vi "ONL.vi"(0 "System no.":i32=1 min=1 max=4 step=1, 2 "Channels to command":string[](array[string]), 3 "Online status":bool=TRUE, 4 "Online status (Array)":bool[](array[boolean]), 5 "error in":errorcluster) -> (19 "error out":errorcluster)   [LabVIEW 2020]
doc: "Switches system online (TRUE) or offline (FALSE). GCS 1.0: Online status is valid for all channels/axes of the system. GCS 2.0: Online status is channel specific.\n\nE-516: Channels to command and Online status (Array) are not valid, use Online status instead to set online status for all channels/axes.\n\nE-517, E-518: Online status is not valid. Use Channels to command and Online status (Array) instead."
uses:
  Communication.llb/Global1.vi
panel:
  # "Switches system online (TRUE) or offline (FALSE). GCS 1.0: Online status is valid for all channels/axes\nof the system. GCS 2.0: Online status is channel specific."
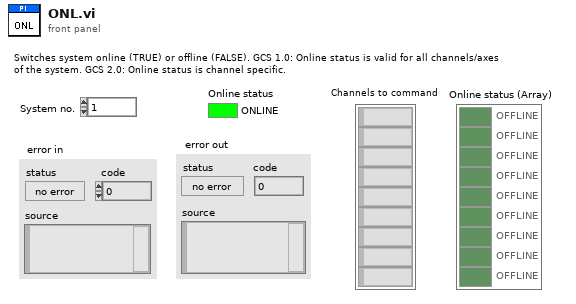
[diagram p1: front panel]
types:
  T1 = typedef "Syntax.ctl" = enum16{"GCS 1.0", "GCS 2.0", "GCS 3.0"}
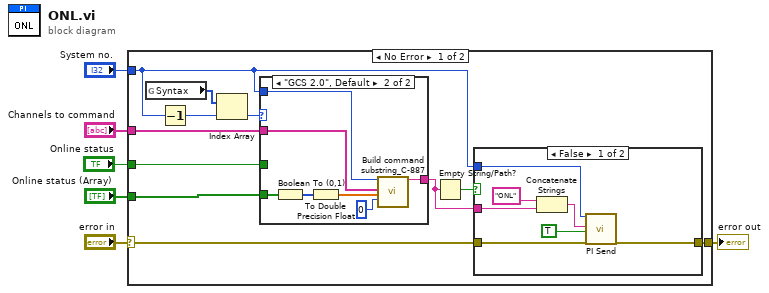
[diagram p0: block diagram]
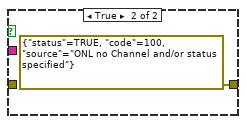
[diagram p2: hidden frame]
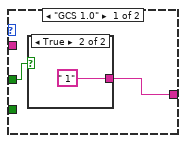
[diagram p3: hidden frame]
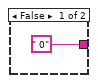
[diagram p4: hidden frame]
diagram:
  n1 = case shown="No Error" "error in" {
    selector: "error in" -> [w7 w37]
    tunnel: "Online status" -> [w17 _]
    tunnel: [w16 w37] -> w5
    tunnel: "Online status (Array)" -> [w12 _]
    tunnel: "Channels to command" -> [w11 _]
    tunnel: "System no." -> [w10 _]
    frame No Error {
      n2 = global read "Global1.vi" "Syntax"() -> (w15:T1[])
      n3 = Decrement(x=w10) -> (x-1=w14:i32)
      n4 = Index Array(array=w15, index=w14) -> (element=w13:T1)
      n5 = case shown="\"GCS 2.0\", Default" w13 {
        tunnel: w17 -> [w27 _]
        tunnel: [w26 w30] -> w9
        tunnel: w12 -> [_ w34]
        tunnel: w11 -> [_ w32]
        tunnel: w10 -> [_ w31]
        frame "GCS 1.0" {
          n6 = case shown="True" w27 {
            tunnel: [" 0" " 1"] -> w26
            frame False {
            }
            frame True {
            }
          }
        }
        frame "GCS 2.0", Default {
          n7 = Boolean To (0,1)(Boolean=w34) -> (0, 1=w35:i16[])
          n8 = To Double Precision Float(number=w35) -> (double precision float=w33:dbl[])
          n9 = call "Build command substring_C-887.vi"("System no."=w31, "Affected axes"=w32, "Parameters"=w33, "No. of digits"=i16 0 ("No.of digits")) -> ("Command substring"=w30:string)  [unwired: 3 in, 12 out]
        }
      }
      n10 = Empty String/Path?(string/path=w9) -> (empty?=w8:bool)
      n11 = case shown="False" w8 {
        tunnel: w7 -> [w24 _]
        tunnel: [w20 errorcluster {"status"=TRUE, "code"=100, "source"="ONL no Channel and/or status specified"} ("error out")] -> w16
        tunnel: w10 -> [w19 _]
        tunnel: w9 -> [w18 _]
        frame False {
          n12 = Concatenate Strings("ONL", w18) -> (w21:string)
          n13 = call "PI Send.vi"("System no."=w19, "String to send"=w21, "Attach termination char.?"=TRUE ("Attach Linefeed?"), "error in"=w24) -> ("error out"=w20:errorcluster)  [unwired: 2 in, 13 out]
        }
        frame True {
        }
      }
    }
    frame Error {
    }
  }
  "error out" <- w5
